vi "DAQ_pp3c_AudioRetriggerDelayConditioning.vi"(0 "Daq config In":T6={"Sound AO"="Dev6/ao0", "Shock intesity AO"="Dev6/ao1", "Code_LED DO"="Dev6/port1:2", "Switch DI"="Dev6/port1/line0", "Webcam"="cam9", "Sound AO task"="", "Sound card task"=0, "Shock intensity AO task"="", "Code_LED DO task"="", "Switch DI task"="", "AO <=> Sound card"=FALSE, "Sound card"=0, "sample rate"=100000.0, "Variable shock"=TRUE, "Webcam on"=FALSE, "Waveform memo"={"t0"=timestamp(0 s since 1904-01-01), "dt"=1.0, "Y"=[]}, "Tone trigger"="PFI1", "Master-9 DO"="", "Master-9 DO task"="Dev6/port0/line5:7", "Master-9 on"=TRUE} {"sample rate" min=8000.0; "Sound card task" format="%.0x"}, 5 "State In":T1={"Curr  tr"=0, "Curr (ms)"=0, "Cum (ms)"=0, "Run loop diff"=0, "Tone countdown (ms)"=0, "Countdown (ms)"=0, "Curr State"=enum."0 NULL", "Prev State"=enum."1 Habituation", "Rw"=FALSE, "Sw"=FALSE, "Tone\nGate"=FALSE, "Punish"=FALSE, "Current DAQ DO Int"=0, "Current Loaded Trial"={"Trial Type Number"=1, "Trial Type"=enum."GO", "Trial Weight"=100, "Shock (mA)"=0.3, "Duration (ms)"=0.25, "Sound Type"=enum."04 FM Sweep", "Stim P1"=4000.0, "Stim P2"=0.0, "Stim P3"=0.0, "Stim P4"=2000.0, "DAQ Amplitude (V)"=0.25}, "Total trials memo"=0, "State start cum memo (ms)"=0, "Last dur jump time memo (ms)"=0, "Last dur shock time memo (ms)"=0, "Tone repeat memo (ms)"=0, "Webcam on"=FALSE, "Webcam recording"=FALSE, "State update flag"=FALSE, "Last loaded shock voltage"=0.0, "Vid upd"=enum."0", "First time tone"=FALSE} {"Current DAQ DO Int" format="%016b"; "Current Loaded Trial"."DAQ Amplitude (V)" min=0.0 max=5.0 format="%_4g"; "Current Loaded Trial"."Shock (mA)" min=-1.0 max=5.0; "Current Loaded Trial"."Trial Weight" step=1; "Current Loaded Trial"."Duration (ms)" min=0.0 max=1.0; "Current Loaded Trial"."Trial Type Number" min=1 max=256 step=1}, 11 "error in (no error)":errorcluster) -> (4 "Daq config Out":T6={"Sound AO"="Dev6/ao0", "Shock intesity AO"="Dev6/ao1", "Code_LED DO"="Dev6/port1:2", "Switch DI"="Dev6/port1/line0", "Webcam"="cam9", "Sound AO task"="", "Sound card task"=0, "Shock intensity AO task"="", "Code_LED DO task"="", "Switch DI task"="", "AO <=> Sound card"=FALSE, "Sound card"=0, "sample rate"=100000.0, "Variable shock"=TRUE, "Webcam on"=FALSE, "Waveform memo"={"t0"=timestamp(0 s since 1904-01-01), "dt"=1.0, "Y"=[]}, "Tone trigger"="PFI1", "Master-9 DO"="", "Master-9 DO task"="Dev6/port0/line5:7", "Master-9 on"=TRUE} {"sample rate" min=8000.0; "Sound card task" format="%.0x"}, 6 "State Out":T1={"Curr  tr"=0, "Curr (ms)"=0, "Cum (ms)"=0, "Run loop diff"=0, "Tone countdown (ms)"=0, "Countdown (ms)"=0, "Curr State"=enum."0 NULL", "Prev State"=enum."1 Habituation", "Rw"=FALSE, "Sw"=FALSE, "Tone\nGate"=FALSE, "Punish"=FALSE, "Current DAQ DO Int"=0, "Current Loaded Trial"={"Trial Type Number"=1, "Trial Type"=enum."GO", "Trial Weight"=100, "Shock (mA)"=0.3, "Duration (ms)"=0.25, "Sound Type"=enum."04 FM Sweep", "Stim P1"=4000.0, "Stim P2"=0.0, "Stim P3"=0.0, "Stim P4"=2000.0, "DAQ Amplitude (V)"=0.25}, "Total trials memo"=0, "State start cum memo (ms)"=0, "Last dur jump time memo (ms)"=0, "Last dur shock time memo (ms)"=0, "Tone repeat memo (ms)"=0, "Webcam on"=FALSE, "Webcam recording"=FALSE, "State update flag"=FALSE, "Last loaded shock voltage"=0.0, "Vid upd"=enum."0", "First time tone"=FALSE} {"Current DAQ DO Int" format="%016b"; "Current Loaded Trial"."DAQ Amplitude (V)" min=0.0 max=5.0 format="%_4g"; "Current Loaded Trial"."Shock (mA)" min=-1.0 max=5.0; "Current Loaded Trial"."Trial Weight" step=1; "Current Loaded Trial"."Duration (ms)" min=0.0 max=1.0; "Current Loaded Trial"."Trial Type Number" min=1 max=256 step=1}, 15 "error out":errorcluster)   [LabVIEW 2013]
uses:
  CTL_pp3c_DaqStatus.ctl
  <vilib>/userdefined/High Color/IMAQdx.ctl
  <vilib>/sound2/lvsound2.llb/Sound Output Task ID.ctl
  CTL_pp3c_LoopState.ctl
  pp3_CTL_BehavioralState.ctl
  pp3_CTL_Trial.ctl
  pp3_CTL_TrialType.ctl
  labolabo2/waveforms/WFTypes.ctl
  <vilib>/sound2/lvsound2.llb/Sound Output Write (DBL Single).vi
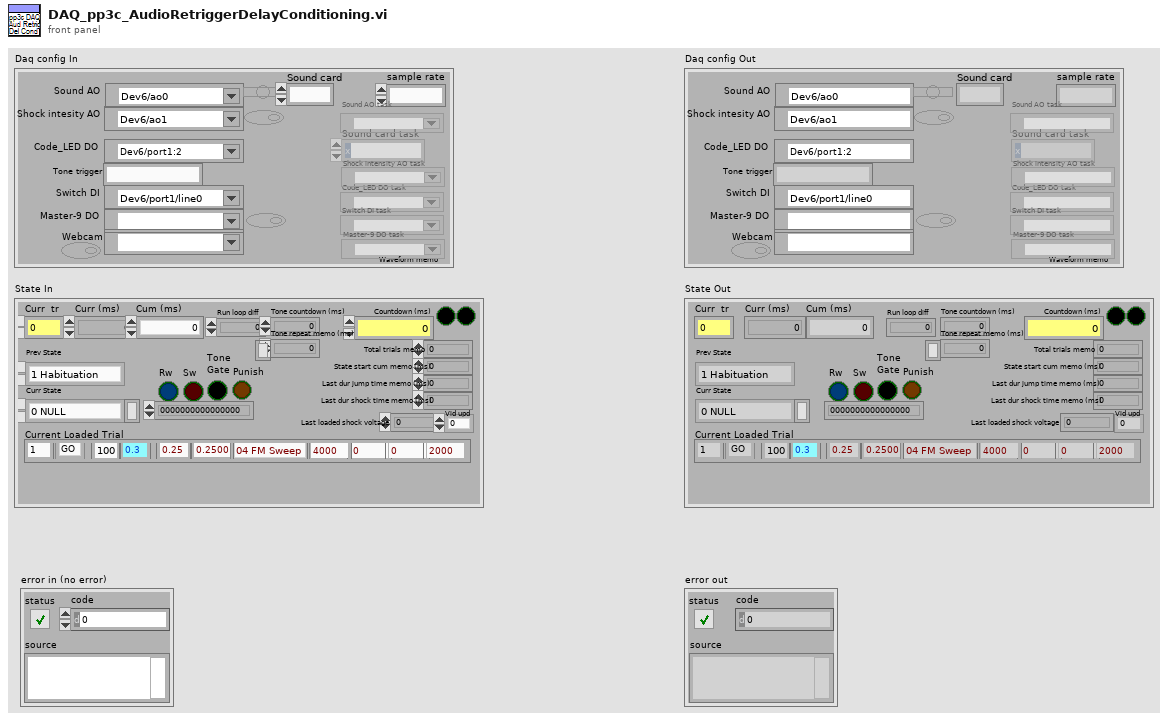
[diagram p1: front panel]
types:
  T1 = typedef "CTL_pp3c_LoopState.ctl" = cluster{"Curr  tr":u16, "Curr (ms)":u32, "Cum (ms)":u64, "Run loop diff":i64, "Tone countdown (ms)":i64, "Countdown (ms)":i64, "Curr State":T2, "Prev State":T2, "Rw":bool, "Sw":bool, "Tone\nGate":bool, "Punish":bool, "Current DAQ DO Int":u16, "Current Loaded Trial":T3, "Total trials memo":i64, "State start cum memo (ms)":i64, "Last dur jump time memo (ms)":i64, "Last dur shock time memo (ms)":i64, "Tone repeat memo (ms)":i64, "Webcam on":bool, "Webcam recording":bool, "State update flag":bool, "Last loaded shock voltage":dbl, "Vid upd":enum16{"0", "1", "2", "3", "4", "5", "6", "7", "8", "9"}, "First time tone":bool}
  T2 = typedef "pp3_CTL_BehavioralState.ctl" = enum8{"0 NULL", "1 Habituation", "2 (Load Trial)", "3 Stay Period", "4 Load Audio/Click Delay", "5 GO Trial", "6 GO Jumped", "7 GO Timeout", "8 NOGO Trial", "9 NOGO Jumped", "10 NOGO Timeout", "11 TEST Trial", "12 TEST Jumped", "13 TEST Timeout", "14 Intertrial Interval", "15 Done"}
  T3 = typedef "pp3_CTL_Trial.ctl" = cluster{"Trial Type Number":i16, "Trial Type":T4, "Trial Weight":u32, "Shock (mA)":dbl, "Duration (ms)":dbl, "Sound Type":T5, "Stim P1":dbl, "Stim P2":dbl, "Stim P3":dbl, "Stim P4":dbl, "DAQ Amplitude (V)":dbl}
  T4 = typedef "pp3_CTL_TrialType.ctl" = enum16{"OFF", "GO", "NOGO", "TEST"}
  T5 = typedef "WFTypes.ctl" = enum16{"00 NULL", "01 DC", "02 Noise", "03 Pure Tone", "04 FM Sweep"}
  T6 = typedef "CTL_pp3c_DaqStatus.ctl" = cluster{"Sound AO":tag, "Shock intesity AO":tag, "Code_LED DO":tag, "Switch DI":tag, "Webcam":T7, "Sound AO task":refnum<k21>, "Sound card task":T8, "Shock intensity AO task":refnum<k21>, "Code_LED DO task":refnum<k21>, "Switch DI task":refnum<k21>, "AO <=> Sound card":bool, "Sound card":u32, "sample rate":dbl, "Variable shock":bool, "Webcam on":bool, "Waveform memo":waveform(dbl), "Tone trigger":string, "Master-9 DO":tag, "Master-9 DO task":refnum<k21>, "Master-9 on":bool}
  T7 = typedef "IMAQdx.ctl" = refnum<k21>
  T8 = typedef "Sound Output Task ID.ctl" = u32
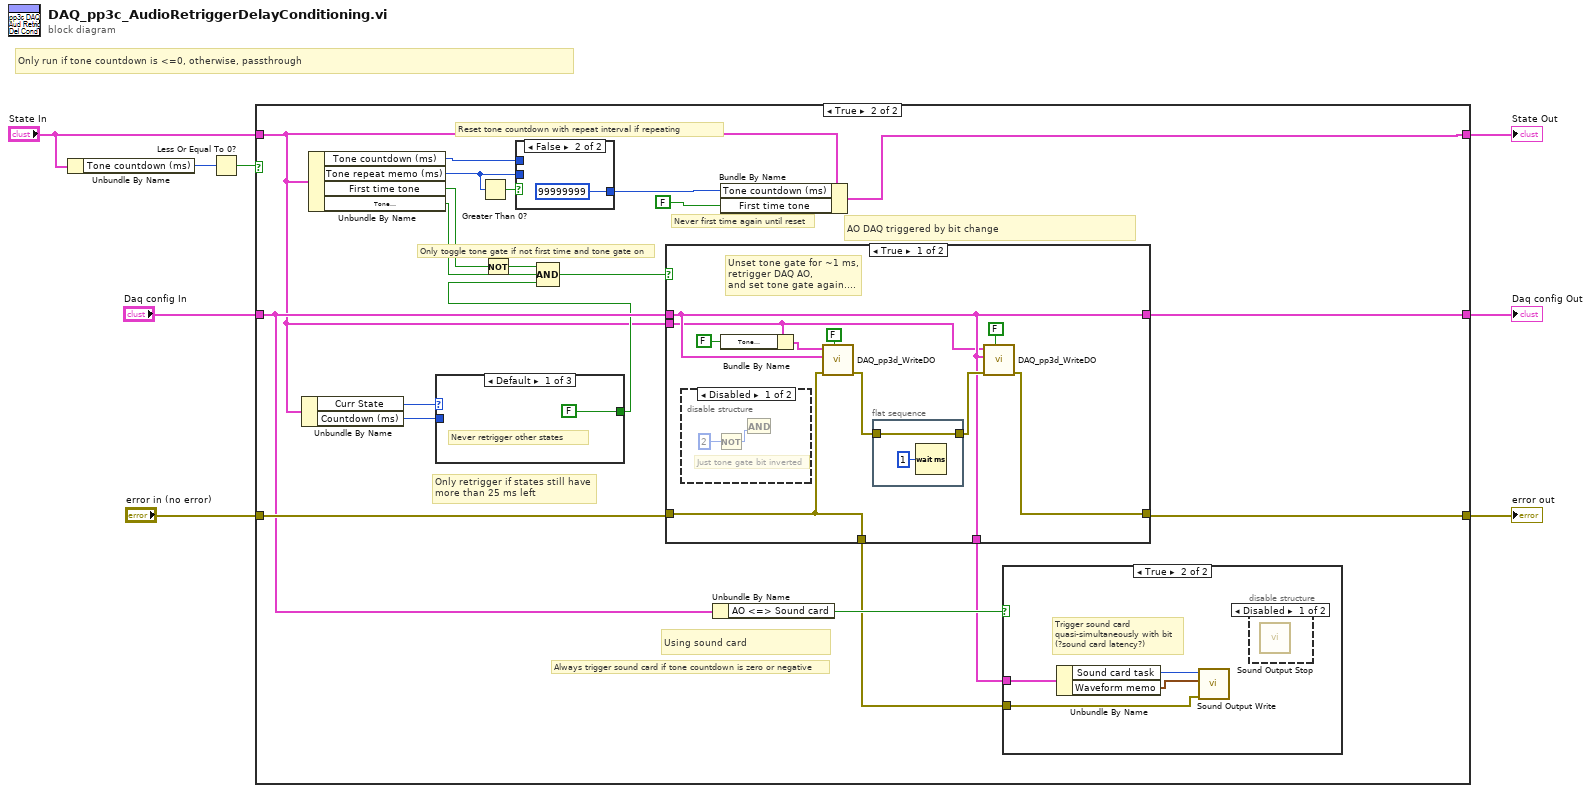
[diagram p0: block diagram]
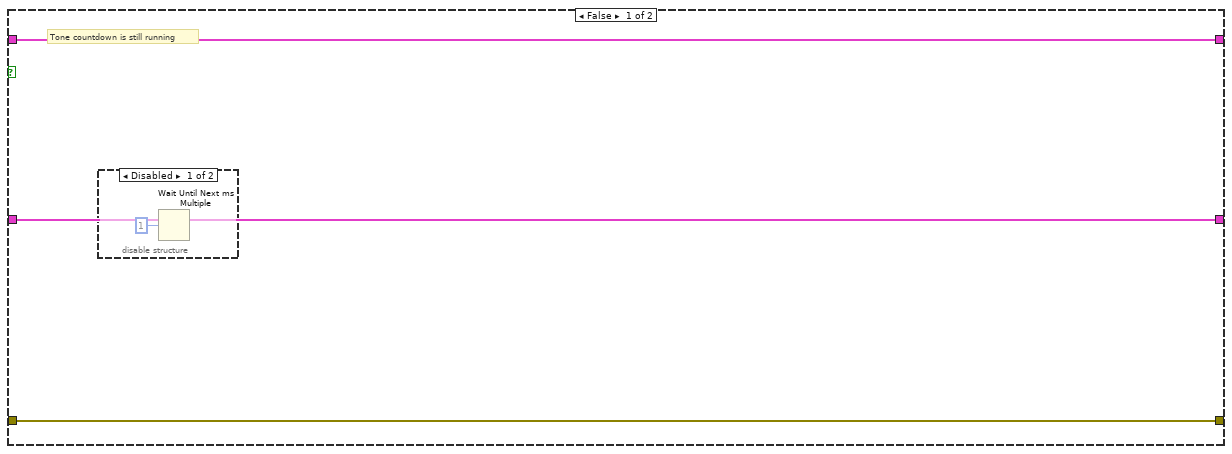
[diagram p2: hidden frame]
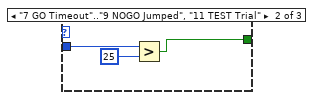
[diagram p6: hidden frame]
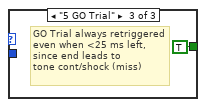
[diagram p7: hidden frame]
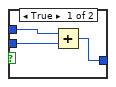
[diagram p10: hidden frame]
diagram:
  # "Only run if tone countdown is <=0, otherwise, passthrough"
  n1 = Unbundle By Name("State In") -> ("Tone countdown (ms)"=w4:i64)
  n2 = Less Or Equal To 0?(x=w4) -> (x <= 0?=w1:bool)
  n3 = case shown="True" w1 {
    tunnel: "Daq config In" -> [w11 w23]
    tunnel: [w11 w31] -> w7
    tunnel: "error in (no error)" -> [w10 w33]
    tunnel: [w10 w32] -> w5
    tunnel: "State In" -> [w9 w13]
    tunnel: [w9 w14] -> w2
    frame False {
      # "Tone countdown is still running"
      n4 = disable-structure shown="Disabled" {
        frame Disabled {
          n5 = Wait Until Next ms Multiple(millisecond multiple=u32 1) -> ()  [unwired: 1 out]
        }
        frame Enabled {
        }
      }
    }
    frame True {
      # "Always trigger sound card if tone countdown is zero or negative"
      # "AO DAQ triggered by bit change"
      # "Using sound card"
      # "Only retrigger if states still have more than 25 ms left"
      # "Never first time again until reset"
      # "Only toggle tone gate if not first time and tone gate on"
      # "Reset tone countdown with repeat interval if repeating"
      n6 = Unbundle By Name(w13) -> ("Curr State"=w21:T2, "Countdown (ms)"=w22:i64)
      n7 = Unbundle By Name(w13) -> ("Tone countdown (ms)"=w29:i64, "Tone repeat memo (ms)"=w30:i64, "First time tone"=w24:bool, "Tone\nGate"=w20:bool)
      n8 = case shown="Default" w21 {
        tunnel: [FALSE w39 TRUE] -> w19
        tunnel: w22 -> [_ w40 _]
        frame Default {
          # "Never retrigger other states"
        }
        frame "7 GO Timeout".."9 NOGO Jumped", "11 TEST Trial" {
          n9 = Greater?(x=w40, y=i64 25) -> (0:w39:bool)
        }
        frame "5 GO Trial" {
          # "GO Trial always retriggered\neven when <25 ms left,\nsince end leads to\ntone cont/shock (miss)"
        }
      }
      n10 = Greater Than 0?(x=w30) -> (x > 0?=w26:bool)
      n11 = Not(x=w24) -> (.not. x?=w25:bool)
      n12 = case shown="False" w26 {
        tunnel: w30 -> [w60 _]
        tunnel: w29 -> [w61 _]
        tunnel: [w59 i64 99999999] -> w28
        frame True {
          n13 = Add(x=w61, y=w60) -> (x+y=w59:i64)
        }
        frame False {
        }
      }
      n14 = Compound Arithmetic op=AND(w25, w20, w19) -> (w27:bool)
      n15 = case shown="True" w27 {
        tunnel: w33 -> [w43 w58]
        tunnel: [w52 w58] -> w32
        tunnel: w23 -> [w48 w57]
        tunnel: [w48 w57] -> w31
        tunnel: [w48 w57] -> w17
        tunnel: [w43 w58] -> w16
        tunnel: w13 -> [w45 _]
        frame True {
          # "Unset tone gate for ~1 ms,\nretrigger DAQ AO,\nand set tone gate again...."
          n16 = disable-structure shown="Disabled" {
            frame Disabled {
              # "Just tone gate bit inverted"
              n17 = Not(x=u16 2) -> (.not. x?=w53:u16)
              n18 = And(y=w53) -> ()  [unwired: 1 in, 1 out]
            }
            frame Enabled {
            }
          }
          n19 = Bundle By Name(cluster=w45, "Tone\nGate"=FALSE ("Tone\nGate")) -> (w46:T1)
          n20 = call "DAQ_pp3d_WriteDO.vi"("Reset to zero"=FALSE, "error in (no error)"=w43, "Daq config"=w48, "State In"=w46) -> ("error out"=w44:errorcluster)  [unwired: 6 in, 1 out]
          n21 = flat-sequence {
            tunnel: [w55] -> w49
            tunnel: w44 -> [w55]
            frame #0 {
              n22 = Wait (ms)(milliseconds to wait=u32 1) -> ()  [unwired: 1 out]
            }
          }
          n23 = call "DAQ_pp3d_WriteDO.vi"("Reset to zero"=FALSE, "error in (no error)"=w49, "Daq config"=w48, "State In"=w45) -> ("error out"=w52:errorcluster)  [unwired: 6 in, 1 out]
        }
        frame False {
        }
      }
      n24 = Unbundle By Name(w23) -> ("AO <=> Sound card"=w18:bool)
      n25 = Bundle By Name(cluster=w13, "Tone countdown (ms)"=w28, "First time tone"=FALSE) -> (w14:T1)
      n26 = case shown="True" w18 {
        tunnel: w17 -> [_ w37]
        tunnel: w16 -> [_ w34]
        frame False {
        }
        frame True {
          # "Trigger sound card\nquasi-simultaneously with bit \n(?sound card latency?)"
          n27 = Unbundle By Name(w37) -> ("Sound card task"=w36:T8, "Waveform memo"=w35:waveform(dbl))
          n28 = call-poly <vilib>:"Sound Output Write.vi"("error in (no error)"=w34, "data"=w35, "task ID"=w36) -> ()  [unwired: 7 in, 2 out]
          n29 = disable-structure shown="Disabled" {
            frame Disabled {
              n30 = call <vilib>:"Sound Output Stop.vi"() -> ()  [unwired: 10 in, 2 out]
            }
            frame Enabled {
            }
          }
        }
      }
    }
  }
  "Daq config Out" <- w7
  "error out" <- w5
  "State Out" <- w2
